vi "Editor UI.vi"(10 "Close Event":refnum<user-event>, 11 "Simulated Scope in":refnum<class "Simulated Scope.lvclass">) -> ()   [LabVIEW 2020, in "Simulated Scope.lvlib" / "Simulated Scope.lvclass"]
uses:
  Simulated Scope.lvclass
  build/ppl/lv-hal.lvlibp/Device/Editor Event Data.ctl
  Simulated Scope.lvclass/Simulated Scope.ctl
  build/ppl/lv-hal.lvlibp/Device/Device.lvclass
  C:/dev/HAL Demo/build/ppl/lv-hal.lvlibp/Device/Device.lvclass
panel:
  in  "Sim Queue Name":string
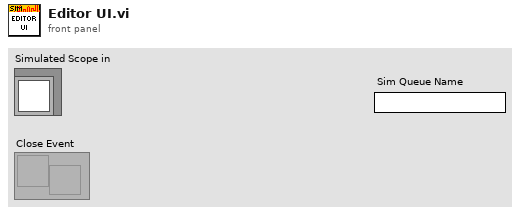
[diagram p1: front panel]
types:
  T1 = typedef "Simulated Scope.lvlib/Simulated Scope.lvclass/Ref Data.ctl" = cluster{"Sim Queue Name":string, "Waveform Queue":refnum<queue>}
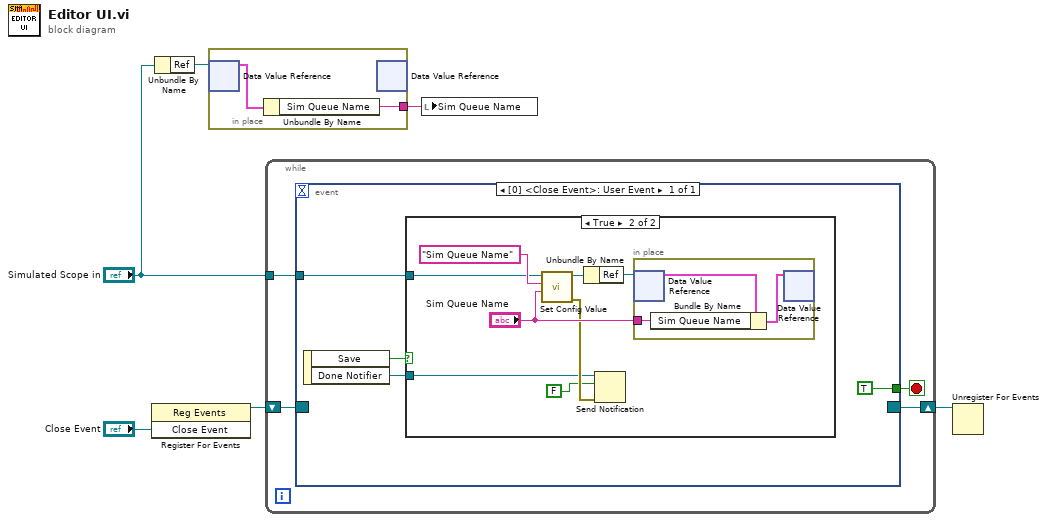
[diagram p0: block diagram]
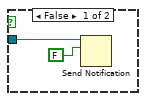
[diagram p2: hidden frame]
diagram:
  n1 = register-events("Close Event") -> (reference out=w3:refnum<event-registration>)  [unwired: 2 in, 1 out]
  n2 = Unbundle By Name("Simulated Scope in") -> ("Ref"=w6:refnum<data-value>)
  n3 = in-place {
    in-place-border: [w7] -> w5
    n4 = in-place-dvr #1(w6) -> (w8:T1)  [unwired: 1 out]
    n5 = Unbundle By Name(w8) -> ("Sim Queue Name"=w7:string)
    n6 = in-place-dvr #1() -> ()  [unwired: 1 in, 2 out]
  }
  n7 = while {
    shift-right: [w11] -> w1
    shift-left: w3 -> [w12]
    tunnel: "Simulated Scope in" -> [w9]
    stop <- w10 stop-if-true
    n8 = event shown="[0] <Close Event>: User Event" {
      selector: w12 -> [_]
      dyn-events: [_] -> w11
      timeout: _ -> [_]
      tunnel: [TRUE] -> w10
      tunnel: w9 -> [w15]
      event User Event {
        n9 = event-data() -> ("Save"=w14:bool, "Done Notifier"=w13:refnum<notifier>)  [unwired: 1 in]
        n10 = case shown="True" w14 {
          tunnel: w15 -> [_ w23]
          tunnel: w13 -> [w18 w20]
          frame False {
            n11 = Send Notification(notification=FALSE, notifier=w18) -> ()  [unwired: 1 in, 2 out]
          }
          frame True {
            n12 = call "Set Config Value.vi"("Value"="Sim Queue Name", "Config Key"="Sim Queue Name", "Device in"=w23) -> ("error out"=w21:errorcluster, "Device out"=w26:refnum<class "Simulated Scope.lvclass">)  [unwired: 7 in]
            n13 = Unbundle By Name(w26) -> ("Ref"=w25:refnum<data-value>)
            n14 = Send Notification(notification=FALSE, notifier=w20, error in (no error)=w21) -> ()  [unwired: 2 out]
            n15 = in-place {
              in-place-border: "Sim Queue Name" -> [w27]
              n16 = in-place-dvr #2(w25) -> (w29:T1)  [unwired: 1 out]
              n17 = Bundle By Name(cluster=w29, "Sim Queue Name"=w27) -> (w28:T1)
              n18 = in-place-dvr #2(w28) -> ()  [unwired: 2 out]
            }
          }
        }
      }
    }
  }
  n19 = local write "Sim Queue Name"(w5) -> ()
  n20 = Unregister For Events(event registration refnum=w1) -> ()  [unwired: 1 in, 1 out]
